vi "Read Both Fans Fault and State.vi"(8 "error in (no error)":errorcluster, 11 "Simulated Dual Fan in":refnum<class "Simulated Dual Fan.lvclass">) -> (0 "error out":errorcluster, 1 "Fan B Fault":bool, 2 "Fan B State":bool, 3 "Fan A Fault":bool, 5 "Fan A State":bool)   [LabVIEW 2018, in "Simulated Dual Fan.lvclass"]
uses:
  Simulated Dual Fan.lvclass
  Cooler Plug-Ins/Simulated Evaporative Cooler.lvclass/Simulation Data_Global.vi
  Cooler Plug-Ins/Simulated Evaporative Cooler.lvclass/Simulated Evaporative Cooler.lvclass
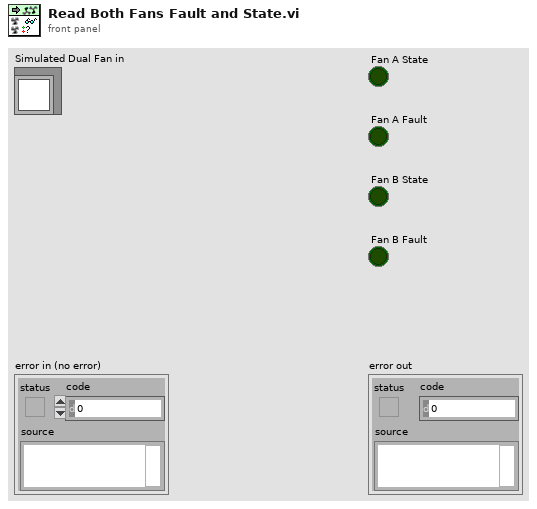
[diagram p1: front panel]
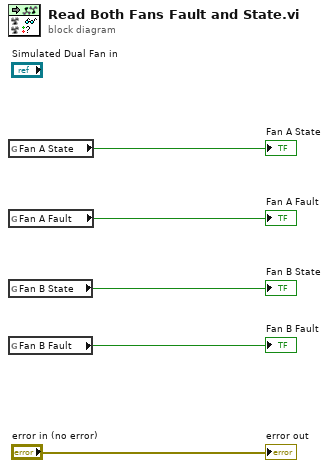
[diagram p0: block diagram]
diagram:
  n1 = global read "Simulation Data_Global.vi" "Fan A State"() -> (→"Fan A State":bool)
  n2 = global read "Simulation Data_Global.vi" "Fan A Fault"() -> (→"Fan A Fault":bool)
  n3 = global read "Simulation Data_Global.vi" "Fan B State"() -> (→"Fan B State":bool)
  n4 = global read "Simulation Data_Global.vi" "Fan B Fault"() -> (→"Fan B Fault":bool)
  "error out" <- "error in (no error)"
